vi "frequencytodt.vi"(10 "Default in":i64, 11 "Frequency":dbl) -> (3 "Default out":i64)   [LabVIEW 2018, in "pid-toolkit.lvlib"]
uses:
  pid-toolkit.lvlib
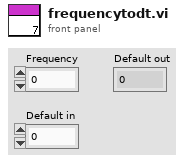
[diagram p1: front panel]
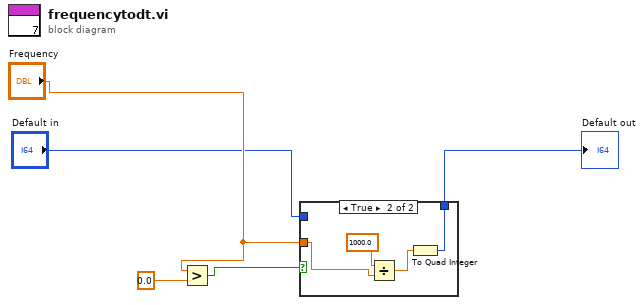
[diagram p0: block diagram]
diagram:
  n1 = Greater?(x="Frequency", y=0.0) -> (0:w4:bool)
  n2 = case shown="True" w4 {
    tunnel: [w6 w8] -> w2
    tunnel: "Default in" -> [w6 _]
    tunnel: "Frequency" -> [_ w7]
    frame False {
    }
    frame True {
      n3 = Divide(x=1000.0, y=w7) -> (x/y=w9:dbl)
      n4 = To Quad Integer(1:w9) -> (0:w8:i64)
    }
  }
  "Default out" <- w2
